vi "Set Focus Index.vi"(8 "error in (no error)":errorcluster, 10 "Focus Index":i8, 11 "Scalable Border in":refnum<class "Scalable Border.lvclass">) -> (0 "error out":errorcluster, 3 "Scalable Border out":refnum<class "Scalable Border.lvclass">)   [LabVIEW 2015, in "Scalable Border.lvclass"]
uses:
  Scalable Border.lvclass
  Scalable Border.lvclass/Scalable Border.ctl
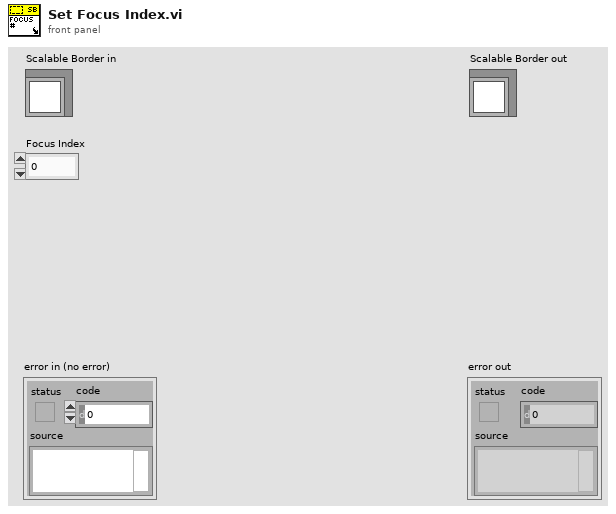
[diagram p1: front panel]
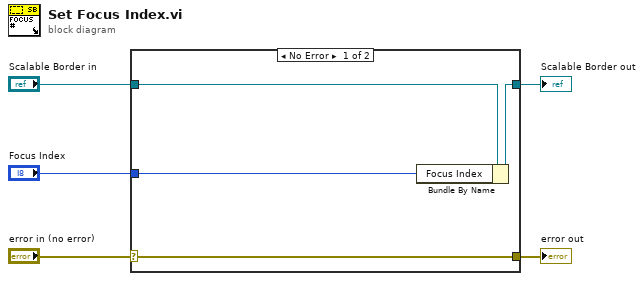
[diagram p0: block diagram]
diagram:
  n1 = case shown="No Error" "error in (no error)" {
    selector: "error in (no error)" -> [w9 w10]
    tunnel: [w9 w10] -> w4
    tunnel: [w7 w11] -> w2
    tunnel: "Scalable Border in" -> [w8 w11]
    tunnel: "Focus Index" -> [w6 _]
    frame No Error {
      n2 = Bundle By Name(cluster=w8, "Focus Index"=w6) -> (w7:refnum<class "Scalable Border.lvclass">)
    }
    frame Error {
    }
  }
  "error out" <- w4
  "Scalable Border out" <- w2
